vi "20TVTI-Change_Sweep_Mode.vi"(8 "error in (no error)":errorcluster, 10 "20TVTI Control":T1, 11 "Mercury Reference In":T2) -> (0 "error out":errorcluster)   [LabVIEW 2019]
uses:
  Equipment/Mercury iXX/Public/Controls/Mercury Reference.ctl
  Equipment/Mercury iXX/Public/Controls/Comms Transport Layer.ctl
  Equipment/Mercury iXX/Private/Controls/Query Dynamic Reference.ctl
  Gustav/20TVTI_Control.ctl
  Equipment/Mercury iXX/Public/Libraries/Temperature/Open/Open Temperature Device.vi
  Equipment/Mercury iXX/Mercury iXX.lvlib
  Equipment/Mercury iXX/Public/Libraries/Temperature.lvlib
  Equipment/Mercury iXX/Public/Libraries/Control Loop.lvlib
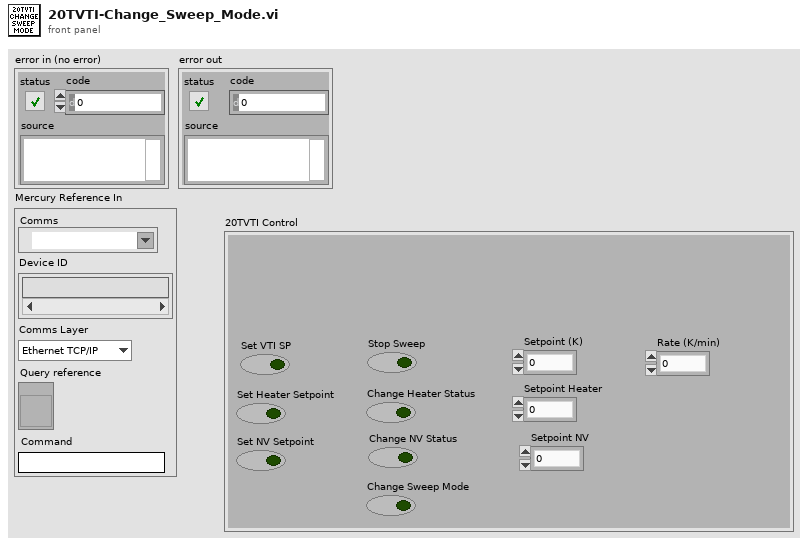
[diagram p1: front panel]
types:
  T1 = typedef "20TVTI_Control.ctl" = cluster{"Set VTI SP":bool, "Change NV Status":bool, "Set NV Setpoint":bool, "Change Heater Status":bool, "Set Heater Setpoint":bool, "Stop Sweep":bool, "Setpoint (K)":dbl, "Rate (K/min)":dbl, "Setpoint Heater":dbl, "Setpoint NV":dbl, "Change Sweep Mode":bool}
  T2 = typedef "Mercury iXX.lvlib/Mercury Reference.ctl" = cluster{"Comms":refnum<visa-resource-name>, "Device ID":string[], "Comms Layer":T3, "Command":string, "Query reference":T4}
  T3 = typedef "Mercury iXX.lvlib/Comms Transport Layer.ctl" = enum16{"Ethernet TCP/IP", "USB", "ISOBus - RS-232", "GPIB"}
  T4 = typedef "Mercury iXX.lvlib/Query Dynamic Reference.ctl" = refnum<vi>
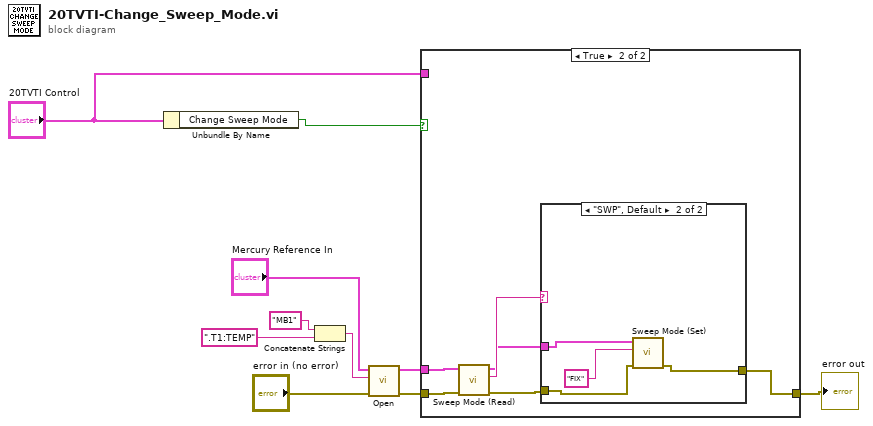
[diagram p0: block diagram]
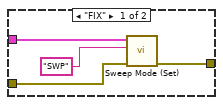
[diagram p3: hidden frame]
diagram:
  n1 = Unbundle By Name("20TVTI Control") -> ("Change Sweep Mode"=w1:bool)
  n2 = Concatenate Strings("MB1", ".T1:TEMP" ("Device Identifier")) -> (w6:string)
  n3 = call-poly "Open.vi"("error in (no error)"="error in (no error)", "Device Identifier"=w6, "Mercury Reference In"="Mercury Reference In") -> ("error out"=w8:errorcluster, "Mercury Reference Out"=w9:T2)  [unwired: 1 in, 6 out]
  n4 = case shown="True" w1 {
    tunnel: w9 -> [_ w17]
    tunnel: w8 -> [w11 w16]
    tunnel: [w11 w12] -> w4
    tunnel: "20TVTI Control" -> [_ _]
    frame False {
    }
    frame True {
      n5 = call "Sweep Mode (Read).vi"("error in"=w16, "Mercury Reference In"=w17) -> ("error out"=w13:errorcluster, "Sweep Mode"=w15:string, "Mercury Reference Out"=w14:T2)  [unwired: 6 in, 1 out]
      n6 = case shown="\"SWP\", Default" w15 {
        tunnel: w14 -> [w20 w25]
        tunnel: w13 -> [w19 w23]
        tunnel: [w18 w22] -> w12
        frame "FIX" {
          n7 = call "Sweep Mode (Set).vi"("error in"=w19, "Sweep Mode"="SWP", "Mercury Reference In"=w20) -> ("error out"=w18:errorcluster)  [unwired: 5 in, 3 out]
        }
        frame "SWP", Default {
          n8 = call "Sweep Mode (Set).vi"("error in"=w23, "Sweep Mode"="FIX", "Mercury Reference In"=w25) -> ("error out"=w22:errorcluster)  [unwired: 5 in, 3 out]
        }
      }
    }
  }
  "error out" <- w4
